vi "close file csv.vi"(11 "file_handle":u32) -> (2 "function return":i32, 3 "file_handle out":u32)   [LabVIEW 2019, in "apdm.lvlib"]
doc: "APDM_EXPORT int apdm_close_file_csv(apdm_csv_t file_handle);"
uses:
  apdm.lvlib
  Lee Lab/CP FES Walking 2018/Code/Working/LabVIEW/apdm.dll
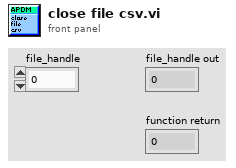
[diagram p1: front panel]
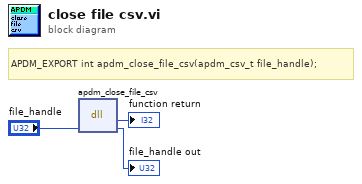
[diagram p0: block diagram]
diagram:
  # "APDM_EXPORT int apdm_close_file_csv(apdm_csv_t file_handle);"
  n1 = dll-call lib="C:/Users/jfalesi/Dropbox/Lee Lab/CP FES Walking 2018/Code/Working/LabVIEW/apdm.*" fn="apdm_close_file_csv"("file_handle"="file_handle") -> (→"function return":i32, "file_handle"=→"file_handle out":u32)  [unwired: 3 in, 2 out]
